vi "Robot Main.vi"() -> ()   [LabVIEW 2017]
doc: "This VI implements the framework and scheduler for your robotics program. It should not be necessary to modify the framework. You are expected to add your code to the VIs called from Robot Main - the ones located in the Team Code folder within the project."
uses:
  <vilib>/Rock Robotics/WPI/Camera/WPI_CameraImageSize.ctl
  PowerUpSrc/TypeDefs/RobotID.ctl
  Robot Global Data.vi
panel:
  out "LoadedRobotID":T1
  in  "Robot ID File":path
  in  "Override Robot ID":bool
  in  "Robot ID":T1
  in  "Image Size":T2=enum."320x240"
  in  "Enable Vision":bool
  in  "Finish":bool
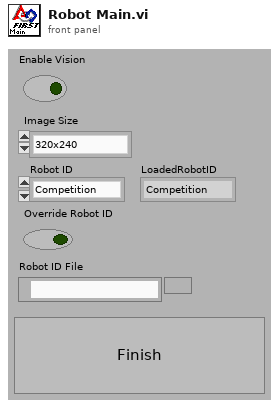
[diagram p1: front panel]
types:
  T1 = typedef "RobotID.ctl" = enum16{"Competition", "Practice", "Programming"}
  T2 = typedef "WPI_CameraImageSize.ctl" = enum16{"640x480", "320x240", "160x120", "Custom"}
  T3 = typedef "Config_Robot.ctl" = cluster{"Motors":cluster{"DriveLeftPrimary":T4, "DriveLeftSecondary1":T4, "DriveRightPrimary":T4, "DriveRightSecondary1":T4, "RightIntake":T4, "LeftIntake":T4, "ArmPivot":T4, "ArmExtend":T4, "ArmPivot2":T4, "Climber":T4}, "Sensors":cluster{"IMU":T7, "LimitSwitch1":T9, "LimitSwitch2":T9, "BeamBreak":T9, "JeVois":T11}, "PID":cluster{"ArmExtend":T13, "ArmRotate":T13, "Drive":T13, "DriveGyro Kp ((in/sec)/deg)":dbl}, "Solenoids":cluster{"ArmClaw":T14, "IntakeExtend":T14, "IntakeOpen":T14, " Shifter":T14}, "RobotDimensions ":T16, "ArmHomePosition":T17}
  T4 = typedef "Config_Motor.ctl" = cluster{"CAN Address":u8, "Invert":bool, "InvertSensor":bool, "Unit Conversion Factor":dbl, "Brake Mode":T5, "Reverse Limt Switch Mode":T6, "Forward Limt Swith Mode":T6}
  T5 = typedef "CTRE_Phoenix_MotorControl_NeutralMode.ctl" = enum8{"EEPROMSetting", "Override to Coast", "Override to Brake"}
  T6 = typedef "CTRE_Phoenix_MotorControl_LimitSwitchNormal.ctl" = enum16{"Normally Open", "Normally Closed", "Disabled"}
  T7 = typedef "Config_IMU.ctl" = cluster{"Yaw Axis":enum16{"X", "Y", "Z"}, "SPI Bus":T8, "AHRS Algorithm":enum16{"Complementary", "Madgwick"}, "Calibration Time (s)":dbl, "Calibrate On Open":bool}
  T8 = typedef "spi_bus.ctl" = enum16{"SPI On-Board, CS0", "SPI On-Board, CS1", "SPI On-Board, CS2", "SPI On-Board, CS3", "SPI MXP", "Invalid"}
  T9 = typedef "Config_DigitalIO.ctl" = cluster{"DIOChannel":T10, "Active Low":bool}
  T10 = typedef "FPGA_DIOChannel.ctl" = enum8{"DIO 0", "DIO 1", "DIO 2", "DIO 3", "DIO 4", "DIO 5", "DIO 6", "DIO 7", "DIO 8", "DIO 9", "DIO MXP 0", "DIO MXP 1", "DIO MXP 2", "DIO MXP 3", "DIO MXP 4", "DIO MXP 5", "DIO MXP 6", "DIO MXP 7", "DIO MXP 8", "DIO MXP 9", "DIO MXP 10", "DIO MXP 11", "DIO MXP 12", "DIO MXP 13", "DIO MXP 14", "DIO MXP 15", "SPI Port CS1", "SPI Port CS2", "SPI Port CS3", "SPI Port MISO", "SPI Port MOSI", "Invalid"}
  T11 = typedef "Config_SerialPort.ctl" = cluster{"Baud Rate":u32, "Parity":u16, "Data Bits":u16, "Stop Bits":u16, "Termination Char (0xA = '\\n' = LF)":u8, "Enable Termination Char? (T)":bool, "Flow Control":u16, "Timeout Value (ms)":u32, "Serial Port":T12}
  T12 = typedef "WPI_SerialPort.ctl" = enum16{"Onboard RS-232", "MXP TTL", "USB 1", "USB 2"}
  T13 = typedef "Config_PIDParams.ctl" = cluster{"P":dbl, "I":dbl, "D":dbl, "F":dbl, "IZone":dbl}
  T14 = typedef "Config_DoubleSolenoid.ctl" = cluster{"Forward Channel":T15, "Invert":bool, "Reverse Channel":T15}
  T15 = typedef "WPI_SolenoidChannel.ctl" = enum8{"Solenoid 0", "Solenoid 1", "Solenoid 2", "Solenoid 3", "Solenoid 4", "Solenoid 5", "Solenoid 6", "Solenoid 7", "Invalid"}
  T16 = typedef "Config_Dimensions.ctl" = cluster{"Length":dbl, "Height":dbl, "HeightOfBumpers":dbl, "DistanceFromFrameEdgeToPyramid ":dbl, "HeightOfFrameToIntake":dbl, "EdgeOfFrameToOrigin":dbl}
  T17 = typedef "Config_ArmHome.ctl" = cluster{"Angle (rad)":dbl, "Radius (in)":dbl}
  T18 = typedef "WPI_DriverStationMatch Info.ctl" = cluster{"Autonomous Elapsed Seconds":dbl, "TeleOp Elapsed Seconds":dbl, "Disabled Elapsed Seconds":dbl, "Visited Autonomous":bool, "Visited TeleOp":bool, "Visited Disabled":bool, "Autonomous Settings":cluster{"Autonomous Style":enum16{"Iterative", "Independent"}, "VI Refnum":refnum<vi>}}
  T19 = typedef "WPI_DriverStationDerivedRobotMode.ctl" = enum16{"Init", "Execute", "Stop"}
  T20 = typedef "WPI_DriverStationRobotMode2.ctl" = enum16{"Autonomous Disabled", "Autonomous Enabled", "Teleop Disabled", "Teleop Enabled", "Disconnected", "Finish", "Test Disabled", "Test Enabled", "Emergency Stopped"}
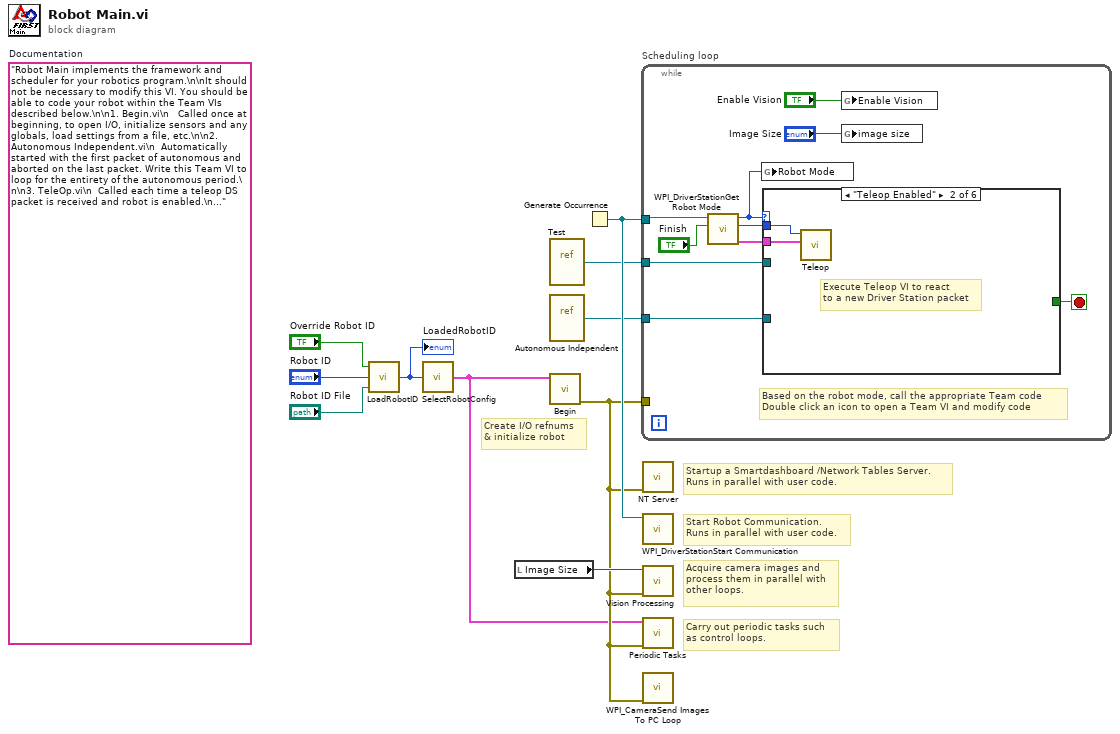
[diagram p0: block diagram]
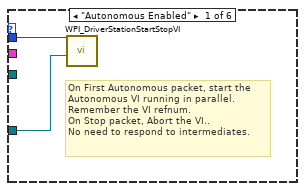
[diagram p2: hidden frame]
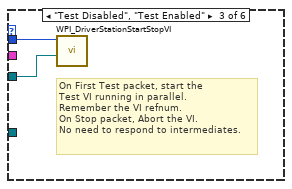
[diagram p3: hidden frame]
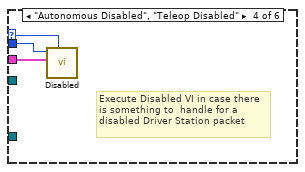
[diagram p4: hidden frame]
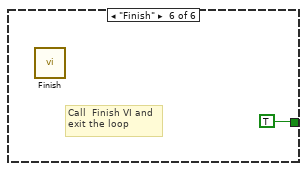
[diagram p6: hidden frame]
diagram:
  (unwired) "Robot Main implements the framework and scheduler for your robotics program.\n\nIt should not be necessary to modify this VI. You should be able to code your robot within the Team VIs described below.\n\n1. Begin.vi\n   Called once at beginning, to open I/O, initialize sensors and any globals, load settings from a file, etc.\n\n2. Autonomous Independent.vi\n  Automatically started with the first packet of autonomous and aborted on the last packet. Write this Team VI to loop for the entirety of the autonomous period.\n\n3. TeleOp.vi\n  Called each time a teleop DS packet is received and robot is enabled.\n\n4. Disabled.vi\n  Called each time a packet is received and the robot is disabled.\n\n5. Test.vi\n  Called Automatically started with the first test packet and aborted on the last. Modify this VI to carry out robot and sensor validation tests.\n\n6. Vision.vi\n  A parallel loop that acquires and processes camera images.\n\n7. PeriodicTasks.vi\n  Parallel loops running at user-defined rates.\n\n8. Finish.vi\n  Called before exiting, so you can save data, clean up I/O, etc.\n"  # Documentation
  # "Startup a Smartdashboard /Network Tables Server.\nRuns in parallel with user code."
  # "Carry out periodic tasks such\nas control loops."
  # "Acquire camera images and\nprocess them in parallel with\nother loops."
  # "Create I/O refnums\n& initialize robot"
  # "Start Robot Communication.\nRuns in parallel with user code."
  n1 = call "LoadRobotID.vi"("Robot ID File"="Robot ID File", "DefaultRobotID"="Robot ID", "OverrideFileValue"="Override Robot ID") -> ("RobotID"=w3:T1)
  "LoadedRobotID" <- w3
  n2 = call "SelectRobotConfig.vi"("Robot ID"=w3) -> ("Selected Config"=w4:T3)
  n3 = local read "Image Size"() -> (w7:T2)
  n4 = vi-ref "Test.vi"() -> (w8:refnum<vi>)
  n5 = vi-ref "Autonomous Independent.vi"() -> (w9:refnum<vi>)
  n6 = call "Begin.vi"("RobotConfig"=w4) -> ("error out"=w6:errorcluster)  [unwired: 1 in, 9 out]
  n7 = Generate Occurrence() -> (w10:refnum<k4>)
  n8 = while "Scheduling loop" {
    tunnel: w10 -> [w19]
    tunnel: w6 -> [_]
    tunnel: w9 -> [w14]
    tunnel: w8 -> [w12]
    stop <- w16 stop-if-true
    # "Based on the robot mode, call the appropriate Team code\nDouble click an icon to open a Team VI and modify code"
    n9 = call <vilib>:"WPI_DriverStationGet Robot Mode.vi"("Finish"="Finish", "DS Occurrence"=w19) -> ("Match Info out"=w17:T18, "Call Context"=w20:T19, "Robot Mode"=w11:T20)  [unwired: 7 out]
    n10 = global write "Robot Global Data.vi" "Robot Mode"(w11) -> ()
    n11 = case shown="\"Teleop Enabled\"" w11 {
      selector: w11 -> [_ _ _ w27 _ _]
      tunnel: w20 -> [w22 w24 w26 w29 _ _]
      tunnel: w17 -> [_ w23 _ w28 _ _]
      tunnel: [_ _ _ _ _ TRUE] -> w16
      tunnel: w14 -> [w21 _ _ _ _ _]
      tunnel: w12 -> [_ _ w25 _ _ _]
      frame "Autonomous Enabled" {
        # "On First Autonomous packet, start the\nAutonomous VI running in parallel.\nRemember the VI refnum.\nOn Stop packet, Abort the VI..\nNo need to respond to intermediates."
        n12 = call <vilib>:"WPI_DriverStationStartStopVI.vi"("VI in"=w21, "Call Context"=w22) -> ()  [unwired: 10 in]
      }
      frame "Teleop Enabled" {
        # "Execute Teleop VI to react\nto a new Driver Station packet"
        n13 = call "Teleop.vi"("Match Info"=w23, "Call Context"=w24) -> ()  [unwired: 1 in, 9 out]
      }
      frame "Test Disabled", "Test Enabled" {
        # "On First Test packet, start the\nTest VI running in parallel.\nRemember the VI refnum.\nOn Stop packet, Abort the VI.\nNo need to respond to intermediates."
        n14 = call <vilib>:"WPI_DriverStationStartStopVI.vi"("VI in"=w25, "Call Context"=w26) -> ()  [unwired: 10 in]
      }
      frame "Autonomous Disabled", "Teleop Disabled" {
        # "Execute Disabled VI in case there\nis something to  handle for a\ndisabled Driver Station packet"
        n15 = call "Disabled.vi"("Robot Mode"=w27, "Match Info"=w28, "Call Context"=w29) -> ()  [unwired: 1 in, 8 out]
      }
      frame "Disconnected", Default {
        # "Driver Station packet didn't arrive.\nPossibly useful for diagnostics"
      }
      frame "Finish" {
        # "Call  Finish VI and\nexit the loop"
        n16 = call "Finish.vi"() -> ()  [unwired: 1 in, 7 out]
      }
    }
    n17 = global write "Robot Global Data.vi" "Enable Vision"("Enable Vision") -> ()
    n18 = global write "Robot Global Data.vi" "image size"("Image Size") -> ()
  }
  n19 = call <vilib>:"NT Server.vi"("error in (no error)"=w6) -> ()  [unwired: 11 in]
  n20 = call <vilib>:"WPI_DriverStationStart Communication.vi"("occurrence"=w10) -> ()  [unwired: 1 in, 10 out]
  n21 = call "Vision Processing.vi"("error in (no error)"=w6, "Image Size"=w7) -> ()  [unwired: 6 out]
  n22 = call "Periodic Tasks.vi"("error in"=w6, "RobotConfig"=w4) -> ()  [unwired: 10 out]
  n23 = call <vilib>:"WPI_CameraSend Images To PC Loop.vi"("error in (no error)"=w6) -> ()  [unwired: 11 in]
